vi "Open Stream (Polymorphic).vi"   [LabVIEW 2015, in "Zaber A Series.lvlib"]
doc: "Opens a stream for receiving coordinated motion commands. \n\nUse zero as the buffer number to open a live steam that will execute commands immediately, or to record commands for later execution specify a buffer number between 1 and the value of the \"stream.numbufs\" setting, which is returned by the Get Stream Support Info VI.\n\nFor a live stream you must specify one or more axis numbers as either integers or strings to execute the commands on. If your device has Firmware version 7, you can use strings and add the word \"lockstep\" before the number to specify an existing lockstep group instead of a single axis. For example \"lockstep 1\" will use lockstep group 1 instead of axis 1.\n\nFor a buffered stream the axis numbers are ignored until you invoke the buffer, but the quantity of them still matters at stream open time.\n\nTo invoke a buffered stream you must open a live stream (and specify the actual axis numbers) and then invoke the buffer using the Call Stream VI.\n\nThis VI does not check in advance for error conditions such as streams not being supported.\n\nThis VI requires that the Initialize VI has been called with the same serial port."
uses:
  Zaber A Series.lvlib
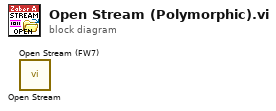
[diagram p0: block diagram]
diagram:
  n1 = call "Open Stream.vi"() -> ()  [unwired: 10 in, 2 out]
  n2 = call "Open Stream (FW7).vi"() -> ()  [unwired: 10 in, 2 out]
